vi "FTPDownloadFile.vi"(8 "error in (no error)":errorcluster, 11 "file":string="FileVersion.txt") -> (0 "error out":errorcluster, 3 "path":path=path "C:/Users/Simon/AppData/Local/Temp/FileVersion.txt")   [LabVIEW 2013, in "main.lvlib"]
uses:
  main.lvlib
panel:
  out "data":string
  out "concatenated string 2":string="ftp -n medimatic.dk"
  out "concatenated string":string="user medimaticftp JAm9Zh71MN\r\nget httpdocs/Content/Upload/FileVersion.txt\r\nbye\r\n"
  in  "User name":string="medimaticftp "
  in  "Password":string="JAm9Zh71MN"
  out "standard output":string
  out "standard error":string
  in  "expected output size  (4096)":u32=4096
  in  "FTP Address":string="medimatic.dk"
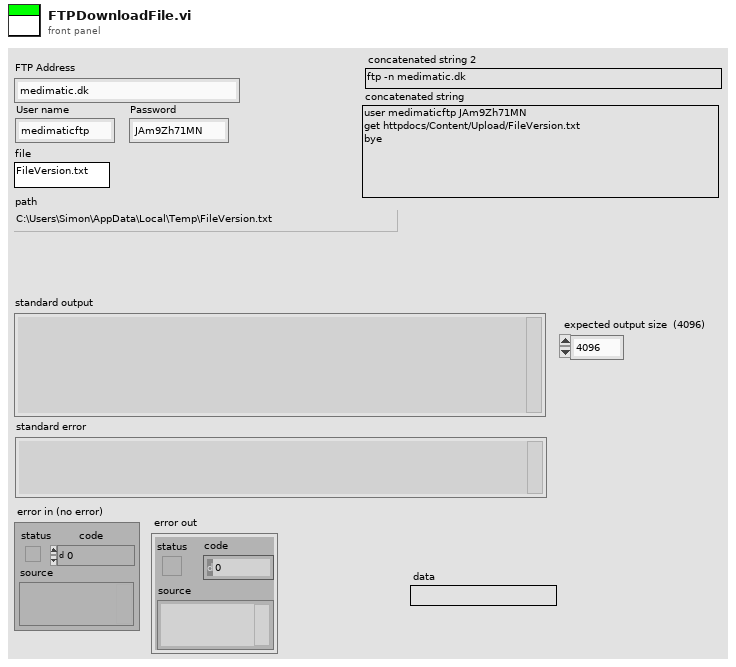
[diagram p1: front panel]
types:
  T1 = enum16{"Read", "Write", "ReadWrite", "BufferedRead", "BufferedReadWrite"}
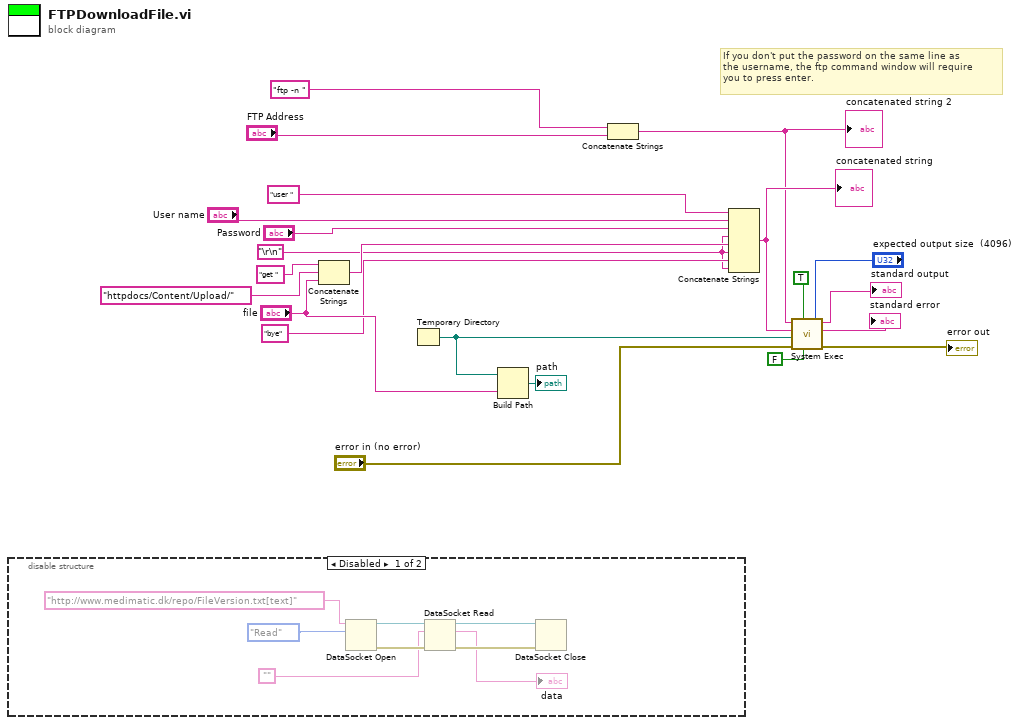
[diagram p0: block diagram]
diagram:
  w1 = "\r\n"
  # "If you don't put the password on the same line as\nthe username, the ftp command window will require \nyou to press enter."
  n1 = disable-structure shown="Disabled" {
    frame Disabled {
      n2 = DataSocket Open(10:T1."Read" ("mode"), 11:"http://www.medimatic.dk/repo/FileVersion.txt[text]" ("URL")) -> (0:w28:errorcluster, 3:w29:refnum<k13>)  [unwired: 2 in]
      n3 = DataSocket Read(8:w28, 10:"", 11:w29) -> (0:w25:errorcluster, 2:→"data":string, 3:w26:refnum<k13>)  [unwired: 2 in, 4 out]
      n4 = DataSocket Close(8:w25, 11:w26) -> ()  [unwired: 1 in, 2 out]
    }
    frame Enabled {
    }
  }
  n5 = Concatenate Strings("get ", "httpdocs/Content/Upload/" ("string"), "file") -> (w5:string)
  n6 = Temporary Directory() -> (w13:path)
  n7 = Build Path(base path=w13, name or relative path="file") -> (appended path=→"path":path)
  n8 = Concatenate Strings("ftp -n " ("command line"), "FTP Address") -> (w8:string)
  "concatenated string 2" <- w8
  n9 = Concatenate Strings("user ", "User name", "Password", w1, w5, w1, "bye", w1) -> (w9:string)
  "concatenated string" <- w9
  n10 = call <vilib>:"System Exec.vi"("expected output size  (4096)"="expected output size  (4096)", "run minimized? (F)"=FALSE, "wait until completion? (T)"=TRUE, "error in (no error)"="error in (no error)", "working directory"=w13, "standard input"=w9, "command line"=w8) -> ("error out"=→"error out":errorcluster, "standard error"=→"standard error":string, "standard output"=→"standard output":string)  [unwired: 1 in, 1 out]
